vi "Wrap.vi"(1 "Current Value in":i32, 8 "max undo steps":i32) -> (15 "Value out":i32)   [LabVIEW 2012]
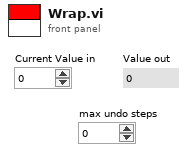
[diagram p1: front panel]
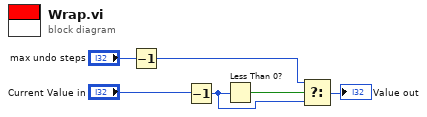
[diagram p0: block diagram]
diagram:
  n1 = Decrement(x="max undo steps") -> (x-1=w2:i32)
  n2 = Decrement(x="Current Value in") -> (x-1=w5:i32)
  n3 = Less Than 0?(x=w5) -> (x < 0?=w6:bool)
  n4 = Select(t=w2, s=w6, f=w5) -> (s? t:f=→"Value out":i32)
